vi "Malleable VIs Basics Lesson 3.vi"() -> ()   [LabVIEW 2023]
doc: "Learn about the type adaptation properties of malleable VIs."
panel:
  out "Last Numeric 5":dbl
  out "Last Numeric 4":dbl
  out "Last Numeric 3":dbl
  out "Last Numeric 2":dbl
  out "Last Error":errorcluster
  out "Last Numeric":dbl
  # "Overview: Learn about the type adaptation properties of malleable VIs.\nInstructions: \n1. Complete the Lesson VIs prior to this one in the Malleable VIs Basics example project.\n2.  Open the block diagram of this VI. Review the lessons presented there."
  # "Note: Browse the diagram of this example to learn about malleable VI concepts. This example is expected to be broken."
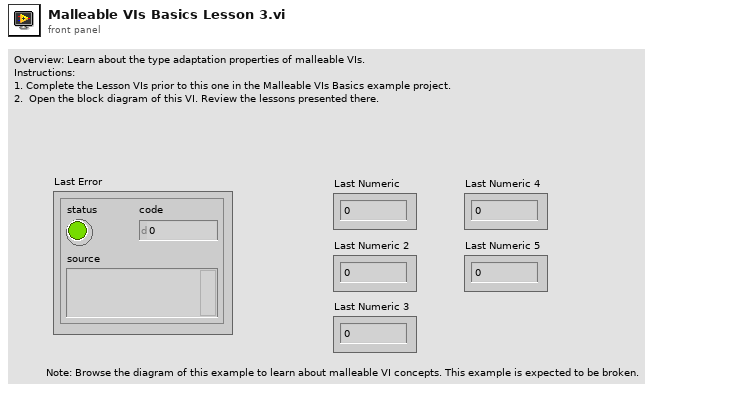
[diagram p1: front panel]
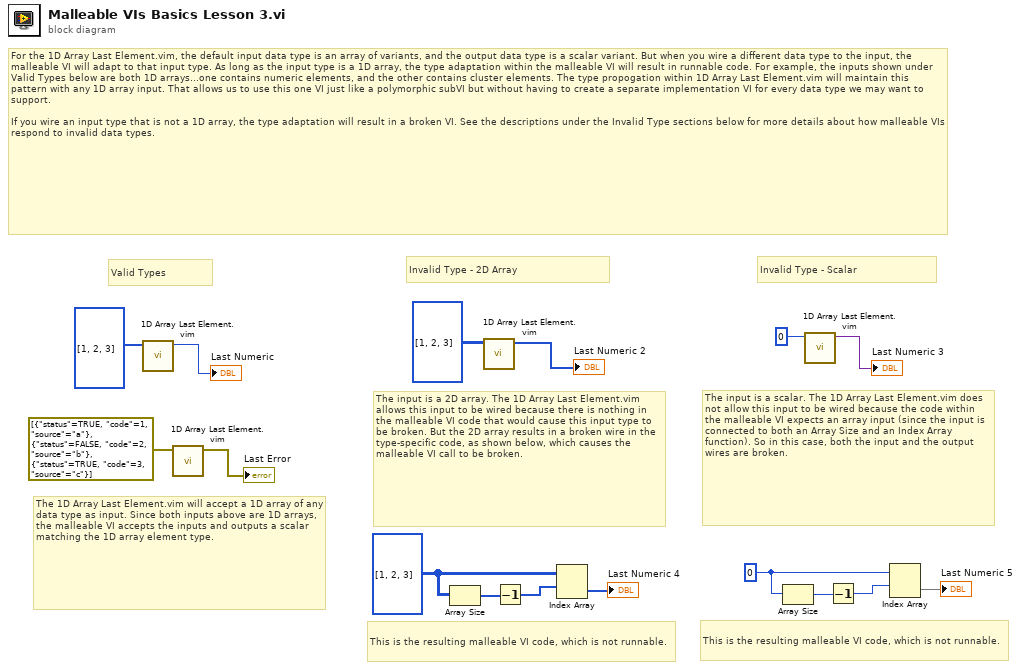
[diagram p0: block diagram]
diagram:
  w9 = 0
  w14 = i32[][] [[1, 2, 3]]
  # "This is the resulting malleable VI code, which is not runnable."
  # "The input is a scalar. The 1D Array Last Element.vim does not allow this input to be wired because the code within the malleable VI expects an array input (since the input is connected to both an Array Size and an Index Array function). So in this case, both the input and the output wires are broken."
  # "This is the resulting malleable VI code, which is not runnable."
  # "Invalid Type - Scalar"
  # "Invalid Type - 2D Array"
  # "Valid Types"
  # "The input is a 2D array. The 1D Array Last Element.vim allows this input to be wired because there is nothing in the malleable VI code that would cause this input type to be broken. But the 2D array results in a broken wire in the type-specific code, as shown below, which causes the malleable VI call to be broken."
  # "The 1D Array Last Element.vim will accept a 1D array of any data type as input. Since both inputs above are 1D arrays, the malleable VI accepts the inputs and outputs a scalar matching the 1D array element type."
  # "For the 1D Array Last Element.vim, the default input data type is an array of variants, and the output data type is a scalar variant. But when you wire a different data type to the input, the malleable VI will adapt to that input type. As long as the input type is a 1D array, the type adaptation within the malleable VI will result in runnable code. For example, the inputs shown under Valid Types below are both 1D arrays...one contains numeric elements, and the other contains cluster elements. The type propogation within 1D Array Last Element.vim will maintain this pattern with any 1D array input. That allows us to use this one VI just like a polymorphic subVI but without having to create a separate implementation VI for every data type we may want to support.\n\nIf you wire an input type that is not a 1D array, the type adaptation will result in a broken VI. See the descriptions under the Invalid Type sections below for more details about how malleable VIs respond to invalid data types."
  n1 = call "1D Array Last Element.vim"("1D Array"=i32[] [1, 2, 3]) -> ("Last Element"=→"Last Numeric":i32)  [unwired: 10 in]
  n2 = call "1D Array Last Element.vim"("1D Array"=errorcluster[] [{"status"=TRUE, "code"=1, "source"="a"}, {"status"=FALSE, "code"=2, "source"="b"}, {"status"=TRUE, "code"=3, "source"="c"}]) -> ("Last Element"=→"Last Error":errorcluster)  [unwired: 10 in]
  n3 = Array Size(array=w14) -> (size(s)=w16:i32[])
  n4 = call "1D Array Last Element.vim"("1D Array"=i32[][] [[1, 2, 3]]) -> ("Last Element"=→"Last Numeric 2":i32[])  [unwired: 10 in]
  n5 = Decrement(x=w16) -> (x-1=w15:i32[])
  n6 = Index Array(array=w14, index (row)=w15) -> (element=→"Last Numeric 4":i32[])  [unwired: 1 in]
  n7 = Array Size(array=w9) -> (size(s)=w10:i32)
  n8 = call "1D Array Last Element.vim"("1D Array"=0) -> ("Last Element"=→"Last Numeric 3":variant)  [unwired: 10 in]
  n9 = Decrement(x=w10) -> (x-1=w11:i32)
  n10 = Index Array(array=w9, index (row)=w11) -> (element=→"Last Numeric 5")  [unwired: 1 in]
